vi "Echo Generator.vi"(1 "回声延时":i32=50, 2 "回声振幅":dbl=0.1 format="%.2f", 3 "频率":dbl=20.0 format="%.2f", 4 "衰减值":dbl=100.0 format="%.2f", 5 "振幅":dbl=1.0 format="%.2f", 6 "采样数":i32=500) -> (0 "回声信号":dbl[](array[numeric]))   [LabVIEW 2014]
uses:
  <vilib>/Analysis/NI_AALPro.lvlib
panel:
  # "回声信号模拟"
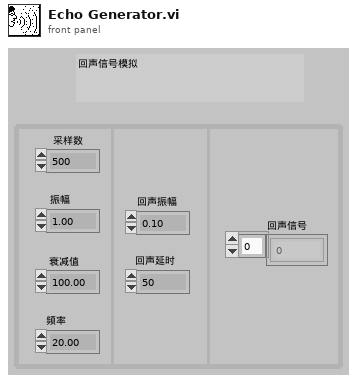
[diagram p1: front panel]
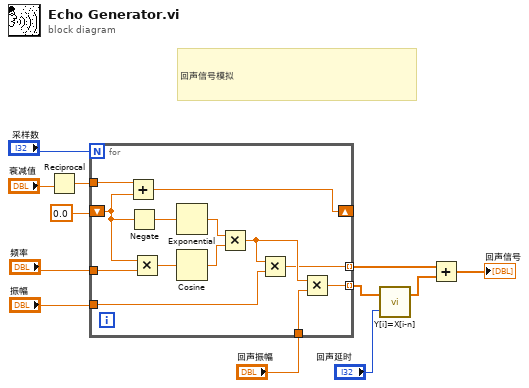
[diagram p0: block diagram]
diagram:
  # "回声信号模拟"
  n1 = Reciprocal(x="衰减值") -> (1/x=w2:dbl)
  n2 = for {
    N: "采样数" -> [_]
    shift-right: [w24] -> _
    shift-left: 0.0 -> [w22]
    tunnel: [w14] -> w9 mode=indexing
    tunnel: [w15] -> w10 mode=indexing
    tunnel: "回声振幅" -> [w16]
    tunnel: "振幅" -> [w18]
    tunnel: "频率" -> [w23]
    tunnel: w2 -> [w25]
    n3 = Add(x=w25, y=w22) -> (x+y=w24:dbl)
    n4 = Negate(x=w22) -> (-x=w13:dbl)
    n5 = Multiply(x=w22, y=w23) -> (x*y=w21:dbl)
    n6 = Exponential(1:w13) -> (0:w19:dbl)
    n7 = Cosine(x=w21) -> (cos(x)=w20:dbl)
    n8 = Multiply(x=w19, y=w20) -> (x*y=w17:dbl)
    n9 = Multiply(x=w17, y=w18) -> (x*y=w14:dbl)
    n10 = Multiply(x=w17, y=w16) -> (x*y=w15:dbl)
  }
  n11 = call <vilib>:"Y[i]=X[i-n].vi"("shifts: n"="回声延时", "Input Array"=w10) -> ("Shifted Array"=w8:dbl[])  [unwired: 1 out]
  n12 = Add(x=w9, y=w8) -> (x+y=→"回声信号":dbl[])
